vi "Passing Arrays as Read-Only ndarrays.vi"() -> ()   [LabVIEW 2020]
uses:
  6d5f1638-640c-4e20-b011-0cee3ae60b95.vi
  688a6956-cd2d-4b8a-a8be-e172edc5432f.vi
  G-Embedded-Python-Interpreter-Toolkit/Null Py Object Refnum.vi
  6d5f1638-640c-4e20-b011-0cee3ae60b95.vi/96ddca92-7bbf-40e2-a1a5-d32f291eb6af.vi
  G-Embedded-Python-Interpreter-Toolkit/Bad Type Error.vi
  G-Embedded-Python-Interpreter-Toolkit/Generate Function Call Argument Info.vi/5ba79b4d-2978-48e4-80f3-d9d30d92ebfd.vi
  688a6956-cd2d-4b8a-a8be-e172edc5432f.vi/6c7a13f1-33d3-431d-8188-904cac5422b3.vi
  G-Embedded-Python-Interpreter-Toolkit/Python Object Reference to Pointer Sized Ref.vi
  G-Embedded-Python-Interpreter-Toolkit/Pointer Sized Ref to Python Object Reference.vi
  G-Embedded-Python-Interpreter-Toolkit/Merge Call Library Errors.vi
  <vilib>/Utility/Data Type/Get Type Information.vi
  <vilib>/Utility/error.llb/Error Cluster From Error Code.vi
  <vilib>/Utility/Data Type/Get Cluster Information.vi
  <vilib>/Utility/Data Type/Get Array Information.vi
  <vilib>/Comparison/Equal/Equal Functor/Equal Functor.lvclass
  G-Embedded-Python-Interpreter-Toolkit/G-Embedded-Python-Interpreter-Toolkit.lvlib
panel:
  out "Average History":dbl(graph)
  out "Sample History":dbl[](graph)
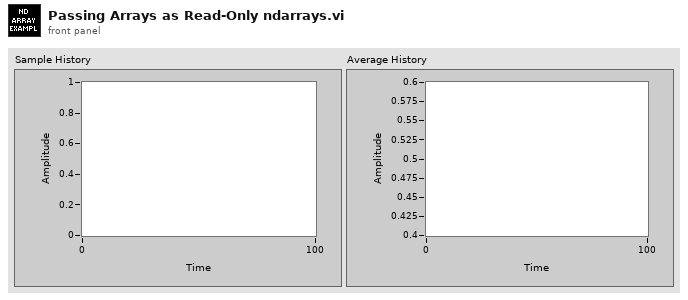
[diagram p1: front panel]
types:
  T1 = typedef "G-Embedded-Python-Interpreter-Toolkit.lvlib/Python Object Reference.ctl" = refnum<k1>
  T2 = typedef "G-Embedded-Python-Interpreter-Toolkit.lvlib/Type Information.ctl" = cluster{"Type":T3, "Array Dimensions":u8}
  T3 = typedef "NI_Data Type.lvlib/Data Type.ctl" = enum8{"Invalid Type", "Void", "I8", "I16", "I32", "I64", "U8", "U16", "U32", "U64", "Single Float", "Double Float", "Extended Float", "Single Complex", "Double Complex", "Extended Complex", "Enum U8", "Enum U16", "Enum U32", "Enum U64", "Single Float With Unit", "Double Float With Unit", "Extended Float With Unit", "Single Complex with Unit", "Double Complex with Unit", "Extended Complex with Unit", "Boolean", "String", "Path", "Picture", "Tag", "Array", "Cluster", "Variant", "LV Variant", "Waveform", "Timestamp", "Digital Waveform", "Digital Data", "ExpressData", "Refnum", "External Data", "VI", "Poly VI", "LabVIEW Class Instance", "Fixed Point", "Set Collection", "Map Collection"}
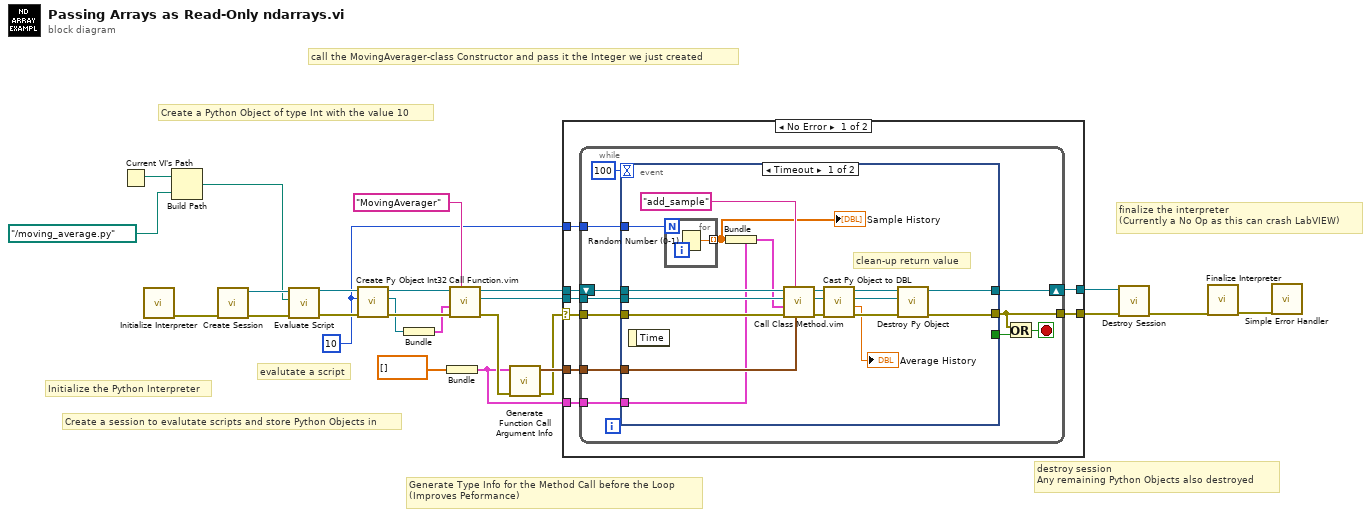
[diagram p0: block diagram]
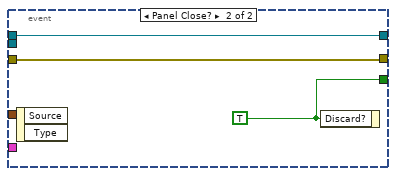
[diagram p2: hidden frame]
diagram:
  w14 = 10 ("Value")
  # "Generate Type Info for the Method Call before the Loop\n(Improves Peformance)"
  # "finalize the interpreter\n(Currently a No Op as this can crash LabVIEW)"
  # "destroy session \nAny remaining Python Objects also destroyed"
  # "Create a Python Object of type Int with the value 10"
  # "call the MovingAverager-class Constructor and pass it the Integer we just created"
  # "evalutate a script"
  # "Create a session to evalutate scripts and store Python Objects in"
  # "Initialize the Python Interpreter"
  n1 = Current VI's Path() -> (path=w22:path)
  n2 = call "Initialize Interpreter.vi"() -> ("error out"=w25:errorcluster)  [unwired: 10 in, 1 out]
  n3 = Build Path(base path=w22, name or relative path=path "../moving_average.py") -> (appended path=w20:path)
  n4 = call "Create Session.vi"("error in (no error)"=w25) -> ("error out"=w24:errorcluster, "Session Handle"=w23:refnum<data-value>)  [unwired: 9 in]
  n5 = call "Evaluate Script.vi"("error in (no error)"=w24, "Script File Path"=w20, "Session Handle in"=w23) -> ("error out"=w17:errorcluster, "Session Handle out"=w18:refnum<data-value>)  [unwired: 7 in]
  n6 = call "Create Py Object Int32.vi"("error in (no error)"=w17, "Value"=w14, "Session Handle in"=w18) -> ("error out"=w16:errorcluster, "Python Object Refnum"=w7:T1, "Session Handle out"=w15:refnum<data-value>)  [unwired: 6 in]
  n7 = Bundle("Python Object Refnum"=w7) -> (w6:cluster{"Python Object Refnum":T1})  [unwired: 1 in]
  n8 = Bundle(dbl[] []) -> (w1:cluster{dbl[]})  [unwired: 1 in]
  n9 = call "Call Function.vim"("Function Name"="MovingAverager", "error in (no error)"=w16, "Arguments in (Default - None)"=w6, "Data Value Reference in"=w15) -> ("error out"=w3:errorcluster, "Returned Python Object Refnum"=w12:T1, "Data Value Reference out"=w13:refnum<data-value>)  [unwired: 5 in]
  n10 = call "Generate Function Call Argument Info.vi"("error in (no error)"=w3, "Data Type"=w1) -> ("error out"=w2:errorcluster, "Array"=w4:T2[])  [unwired: 8 in]
  n11 = case shown="No Error" w2 {
    selector: w2 -> [w33 w68]
    tunnel: w14 -> [w27 _]
    tunnel: w13 -> [w32 w67]
    tunnel: w12 -> [w31 _]
    tunnel: [w30 w68] -> w11
    tunnel: [w29 w67] -> w10
    tunnel: w4 -> [w28 _]
    tunnel: w1 -> [w26 _]
    frame No Error {
      n12 = while {
        tunnel: w33 -> [w44]
        shift-right: [w40] -> w29
        shift-left: w32 -> [w43]
        tunnel: w31 -> [w42]
        tunnel: [w38] -> w30
        tunnel: w28 -> [w37]
        tunnel: w27 -> [w36]
        tunnel: w26 -> [w35]
        stop <- w41 stop-if-true
        n13 = event shown="[0] Timeout" {
          selector: _ -> [_ _]
          dyn-events: _ -> [_ _]
          timeout: 100 -> [_ _]
          tunnel: w44 -> [w62 w66]
          tunnel: w43 -> [w61 w65]
          tunnel: w42 -> [w60 _]
          tunnel: [w52 w66] -> w38
          tunnel: [w51 w65] -> w40
          tunnel: [_ w64] -> w39
          tunnel: w37 -> [w50 _]
          tunnel: w36 -> [w49 _]
          tunnel: w35 -> [w46 _]
          event Timeout {
            # "clean-up return value"
            n14 = event-data() -> ()  [unwired: 1 in, 1 out]
            n15 = for {
              N: w49 -> [_]
              tunnel: [w63] -> w47 mode=indexing
              n16 = Random Number (0-1)() -> (number: 0 to 1=w63:dbl)
            }
            "Sample History" <- w47
            n17 = Bundle(cluster=w46, w47) -> (w48:cluster{dbl[]})
            n18 = call "Call Class Method.vim"("Args Cluster Type Info (Empty - Generate)"=w50, "Function Name"="add_sample", "error in (no error)"=w62, "Arguments in (Default - Empty)"=w48, "Class Instance"=w60, "Data Value Reference in"=w61) -> ("error out"=w58:errorcluster, "Returned Python Object Refnum"=w56:T1, "Data Value Reference out"=w57:refnum<data-value>)  [unwired: 3 in]
            n19 = call "Cast Py Object to DBL.vi"("error in (no error)"=w58, "Python Object Refnum in"=w56, "Session Handle in"=w57) -> ("error out"=w53:errorcluster, "Value"=→"Average History":dbl, "Python Object Refnum out"=w54:T1, "Session Handle out"=w55:refnum<data-value>)  [unwired: 5 in]
            n20 = call "Destroy Py Object.vi"("error in (no error)"=w53, "Python Object Refnum"=w54, "Session Handle in"=w55) -> ("error out"=w52:errorcluster, "Session Handle out"=w51:refnum<data-value>)  [unwired: 7 in]
          }
          event Panel Close? {
            w64 = TRUE ("Discard?")
            n21 = event-data() -> ()  [unwired: 1 in, 2 out]
            n22 = event-data("Discard?"=w64) -> ()  [unwired: 1 in, 1 out]
          }
        }
        n23 = Or(x=w38, y=w39) -> (x .or. y?=w41:bool)
      }
    }
    frame Error {
    }
  }
  n24 = call "Destroy Session.vi"("error in (no error)"=w11, "Session Handle"=w10) -> ("error out"=w9:errorcluster)  [unwired: 9 in]
  n25 = call "Finalize Interpreter.vi"("error in (no error)"=w9) -> ("error out"=w8:errorcluster)  [unwired: 10 in]
  n26 = call <vilib>:"Simple Error Handler.vi"("error in (no error)"=w8) -> ()  [unwired: 4 in, 5 out]
